vi "zmq threadclose.vi"(8 "error in (no error)":errorcluster, 11 "thread_":u32) -> (0 "error out":errorcluster, 3 "thread_ out":u32)   [LabVIEW 2025, in "LibZMQ.lvlib"]
doc: "ZMQ_EXPORT void zmq_threadclose (void *thread_);"
uses:
  LibZMQ.lvlib
  LV/LibZMQ/libzmq/lv_x86/bin/Release/libzmq-v143-mt-4_3_6.dll
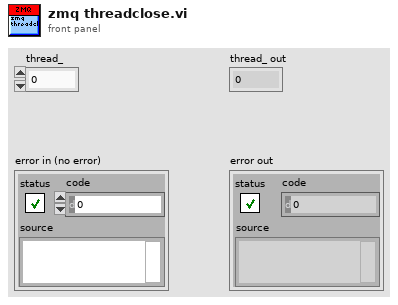
[diagram p1: front panel]
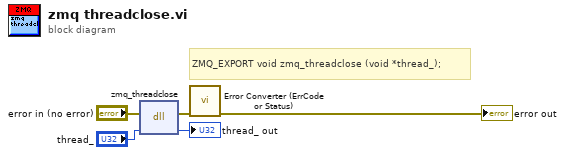
[diagram p0: block diagram]
diagram:
  # "ZMQ_EXPORT void zmq_threadclose (void *thread_);"
  n1 = dll-call lib="C:/LV/LibZMQ/libzmq/lv_x86/bin/Release/libzmq-v143-mt-4_3_6.*" fn="zmq_threadclose"(error in="error in (no error)", "thread_"="thread_") -> (error out=w2:errorcluster, "thread_"=→"thread_ out":u32)  [unwired: 3 in, 1 out]
  n2 = call "Error Converter (ErrCode or Status).vi"("error in (no error)"=w2) -> ("error out"=→"error out":errorcluster)  [unwired: 10 in]
